vi "refocus.vi"() -> ()   [LabVIEW 2022 SP3]
panel:
  in  "error in (no error)":errorcluster
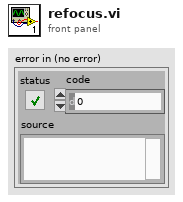
[diagram p1: front panel]
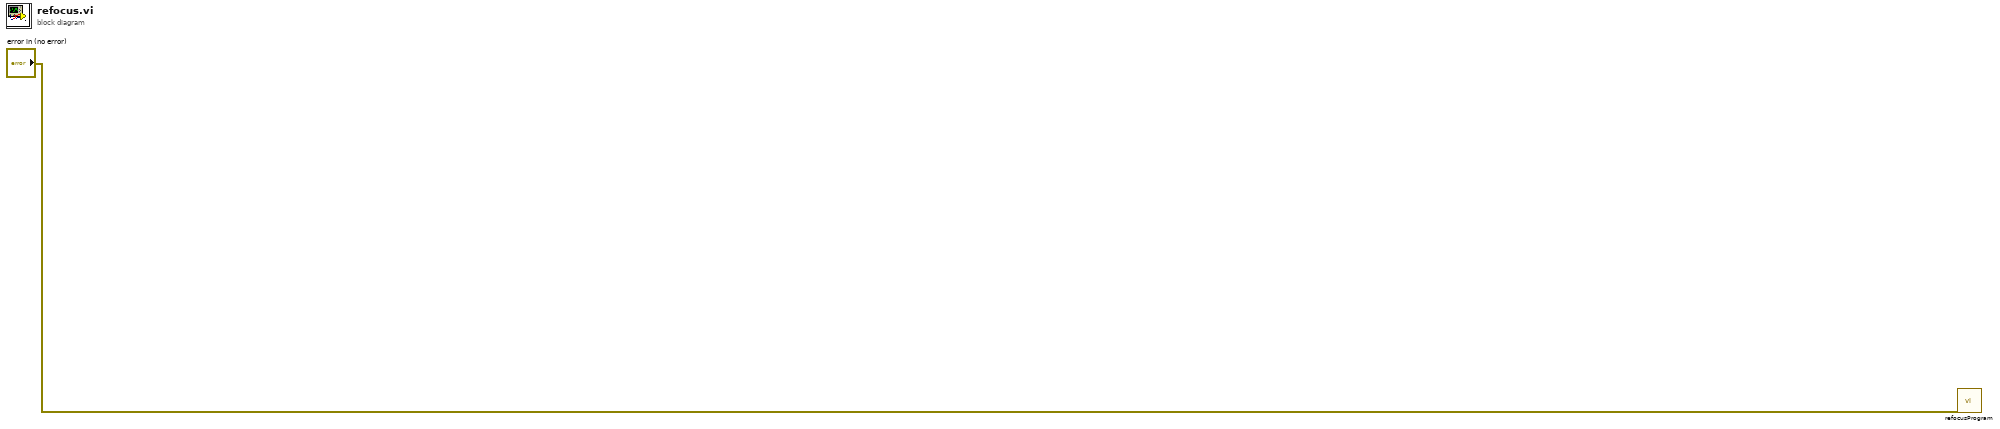
[diagram p0: block diagram]
diagram:
  n1 = call "refocusProgram.vi"("error in (no error)"="error in (no error)") -> ()  [unwired: 11 in]
